vi "User Current Output_Buffer_Dbl_VIG.vi"(7 "Operation":enum16{"get data", "set data", "initialize"}(ring)=enum."set data", 8 "error in":errorcluster, 11 "Numeric":dbl) -> (0 "error out":errorcluster, 3 "Numeric":dbl)   [LabVIEW 2018]
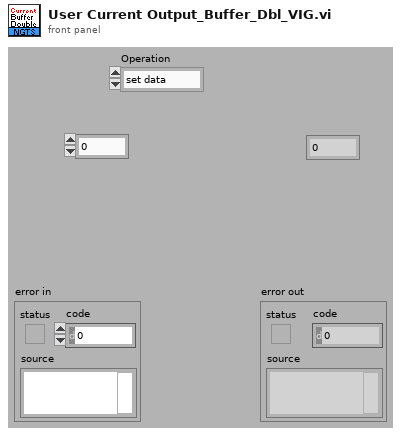
[diagram p1: front panel]
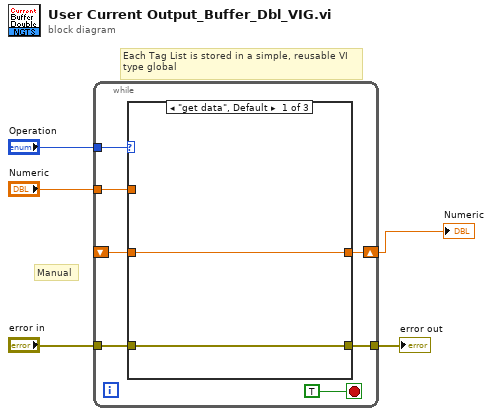
[diagram p0: block diagram]
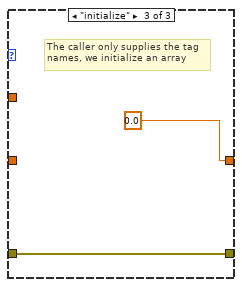
[diagram p3: hidden frame]
diagram:
  # "Manual"
  # "Each Tag List is stored in a simple, reusable VI\ntype global"
  n1 = while {
    tunnel: "Operation" -> [w12]
    tunnel: "Numeric" -> [w10]
    tunnel: "error in" -> [w9]
    tunnel: [w8] -> w2
    shift-right: [w7] -> w1
    shift-left: _ -> [w6]
    stop <- TRUE stop-if-true
    n2 = case shown="\"get data\", Default" w12 {
      tunnel: w10 -> [_ w15 _]
      tunnel: w9 -> [w14 w16 w18]
      tunnel: [w14 w16 w18] -> w8
      tunnel: [w13 w15 0.0 ("element")] -> w7
      tunnel: w6 -> [w13 _ _]
      frame "get data", Default {
      }
      frame "set data" {
      }
      frame "initialize" {
        # "The caller only supplies the tag\nnames, we initialize an array"
      }
    }
  }
  "error out" <- w2
  "Numeric" <- w1
